vi "Marker Notch Search Result.vi"(8 "error in (no error)":errorcluster, 9 "Marker (1)":i32=1, 10 "Channel (1)":i32=1, 11 "VISA resource name":refnum<visa-resource-name>) -> (0 "error out":errorcluster, 1 "Q Value":dbl, 2 "Center Frequency":dbl, 3 "VISA resource name out":refnum<visa-resource-name>, 4 "Loss":dbl, 5 "Bandwidth":dbl)   [LabVIEW 2020, in "Agilent ENA Series.lvlib"]
doc: "Reads out the notch search result of selected marker, for the active trace of selected channel.\n\nNotes:\n(1) This VI is not supported by E5070B, E5071B, E5080A, E5080B"
uses:
  <instrlib>/Agilent ENA Series/Agilent ENA Series.lvlib
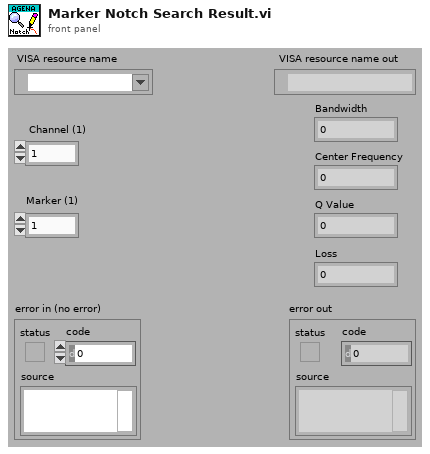
[diagram p1: front panel]
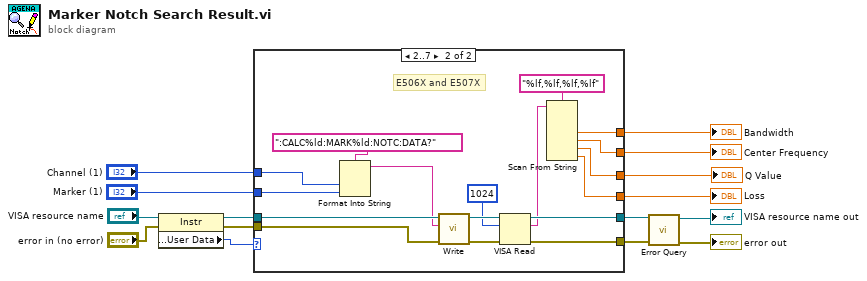
[diagram p0: block diagram]
diagram:
  n1 = property class="Instr"(reference="VISA resource name", error in="error in (no error)") -> (reference out=w15:refnum<visa-resource-name>, error out=w14:errorcluster, "General Settings:User Data"=w9:u32)
  n2 = case shown="2..7" w9 {
    tunnel: w15 -> [w17 w34]
    tunnel: w14 -> [w16 w33]
    tunnel: [w17 w29] -> w4
    tunnel: [w16 w28] -> w3
    tunnel: "Channel (1)" -> [_ w27]
    tunnel: "Marker (1)" -> [_ w26]
    tunnel: [_ w21] -> w8
    tunnel: [_ w20] -> w7
    tunnel: [_ w19] -> w6
    tunnel: [_ w18] -> w5
    frame 0, Default {
    }
    frame 2..7 {
      # "E506X and E507X"
      n3 = Format Into String(format string=":CALC%ld:MARK%ld:NOTC:DATA?", w27, w26) -> (resulting string=w24:string)  [unwired: 2 in, 1 out]
      n4 = call <instrlib>:"Write.vi"("error in (no error)"=w33, "String ()"=w24, "VISA resource name"=w34) -> ("error out"=w31:errorcluster, "VISA resource name out"=w32:refnum<visa-resource-name>)  [unwired: 6 in, 1 out]
      n5 = VISA Read(VISA resource name=w32, byte count=u32 1024, error in (no error)=w31) -> (VISA resource name out=w29:refnum<visa-resource-name>, read buffer=w22:string, error out=w28:errorcluster)  [unwired: 1 out]
      n6 = Scan From String(format string="%lf,%lf,%lf,%lf", input string=w22) -> (output 1=w21:dbl, output 2=w20:dbl, output 3=w19:dbl, output 4=w18:dbl)  [unwired: 6 in, 3 out]
    }
  }
  "Bandwidth" <- w8
  "Center Frequency" <- w7
  "Q Value" <- w6
  "Loss" <- w5
  n7 = call <instrlib>:"Error Query.vi"("error in (no error)"=w3, "VISA resource name"=w4) -> ("error out"=→"error out":errorcluster, "VISA resource name out"=→"VISA resource name out":refnum<visa-resource-name>)  [unwired: 6 in, 2 out]
